vi "Permissions to Bit Mask.vi"(1 "Permissions":T1) -> (0 "Bit Mask":i32)   [LabVIEW 2017, in "Toolkit.lvlib" / "SFTP File.lvclass"]
uses:
  SFTP File.lvclass
  API/Typedefs/Permissions.ctl
  API/Typedefs/Modes.ctl
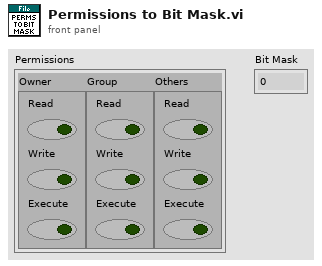
[diagram p1: front panel]
types:
  T1 = typedef "Toolkit.lvlib/SFTP File.lvclass/Permissions.ctl" = cluster{"Owner":T2, "Group":T2, "Others":T2}
  T2 = typedef "Toolkit.lvlib/SFTP File.lvclass/Modes.ctl" = cluster{"Read":bool, "Write":bool, "Execute":bool}
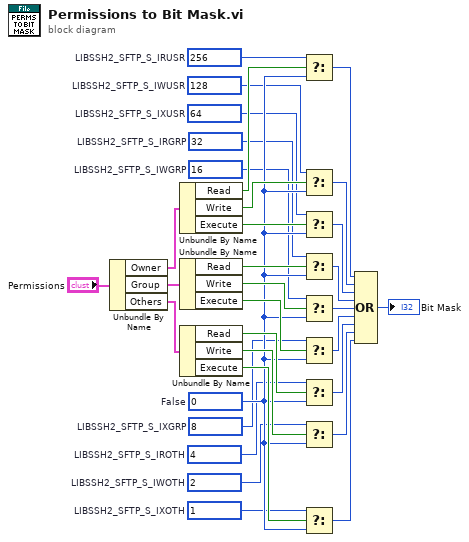
[diagram p0: block diagram]
diagram:
  w1 = 1  # LIBSSH2_SFTP_S_IXOTH
  w2 = 2  # LIBSSH2_SFTP_S_IWOTH
  w3 = 4  # LIBSSH2_SFTP_S_IROTH
  w4 = 8  # LIBSSH2_SFTP_S_IXGRP
  w5 = 16  # LIBSSH2_SFTP_S_IWGRP
  w6 = 32  # LIBSSH2_SFTP_S_IRGRP
  w7 = 64  # LIBSSH2_SFTP_S_IXUSR
  w8 = 128  # LIBSSH2_SFTP_S_IWUSR
  w9 = 256  # LIBSSH2_SFTP_S_IRUSR
  w20 = 0  # False
  n1 = Unbundle By Name("Permissions") -> ("Owner"=w32:T2, "Group"=w31:T2, "Others"=w30:T2)
  n2 = Unbundle By Name(w32) -> ("Read"=w29:bool, "Write"=w28:bool, "Execute"=w27:bool)
  n3 = Unbundle By Name(w31) -> ("Read"=w26:bool, "Write"=w25:bool, "Execute"=w24:bool)
  n4 = Unbundle By Name(w30) -> ("Read"=w23:bool, "Write"=w22:bool, "Execute"=w21:bool)
  n5 = Select(t=w9, s=w29, f=w20) -> (s? t:f=w19:i32)
  n6 = Select(t=w8, s=w28, f=w20) -> (s? t:f=w18:i32)
  n7 = Select(t=w7, s=w27, f=w20) -> (s? t:f=w17:i32)
  n8 = Select(t=w6, s=w26, f=w20) -> (s? t:f=w16:i32)
  n9 = Select(t=w5, s=w25, f=w20) -> (s? t:f=w15:i32)
  n10 = Select(t=w4, s=w24, f=w20) -> (s? t:f=w14:i32)
  n11 = Select(t=w3, s=w23, f=w20) -> (s? t:f=w13:i32)
  n12 = Select(t=w2, s=w22, f=w20) -> (s? t:f=w12:i32)
  n13 = Select(t=w1, s=w21, f=w20) -> (s? t:f=w11:i32)
  n14 = Compound Arithmetic op=OR(w19, w18, w17, w16, w15, w14, w13, w12, w11) -> (→"Bit Mask":i32)
